vi "shuttercontrol.vi"(1 "error in":errorcluster, 2 "command":string) -> (0 "error out":errorcluster)   [LabVIEW 2015]
uses:
  <vilib>/DAQmx/write.llb/DAQmx Write (Digital Bool 1Line 1Point).vi
  <vilib>/DAQmx/create/channels.llb/DAQmx Create Channel (DO-Digital Output).vi
  <vilib>/DAQmx/miscellaneous.llb/DAQmx Fill In Error Info.vi
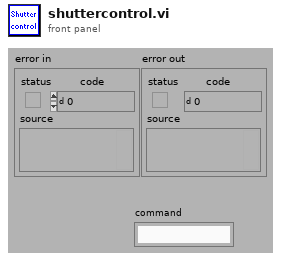
[diagram p1: front panel]
types:
  T1 = typedef "XYZStage.lvlib/XYZStage Configuration.ctl" = cluster{"VISA resource name":refnum<visa-resource-name>, "Timeout (3sec)":u32}
  T2 = cluster{"StageS":i32, "StageL":i32, "currmeas data dir":path, "image OD":u16, "contour OD":u16, "point OD":u16, "AOlines":tag[], "AIlines":tag[], "CI lines":tag[], "DO lines":tag[], "AO names":string[], "CI names":string[], "AI names":string[], "DO names":string[], "CIextensions":string[], "AIextensions":string[], "Voltage to Ygalvo":i32, "Voltage to Xgalvo":i32, "Voltage to patch":i32, "640 shutter":i32, "2P shutter":i32, "LT timestamp":u32, "Vp":i32, "Ip":i32, "camera trigger":i32, "master data dir":path, "voltage to Zpos":i32, "Vto2P":i32, "640 AO":i32, "488 AO":i32, "532 AO":i32, "640TTL":u32, "488TTL":u32, "532TTL":u32, "Device 1 sampleclock out":tag, "Device 1 Starttrigger out":tag, "Device 2 sampleclock in":tag, "Device 2 StartTrigger in ":tag, "2PODTTL":u32, "488 shutter":u32, "LCVR red":u32, "LCVR blue":u32, "Sutter Stage Config":T1}
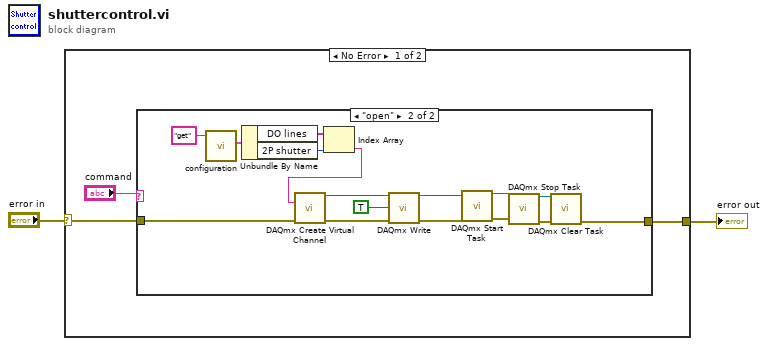
[diagram p0: block diagram]
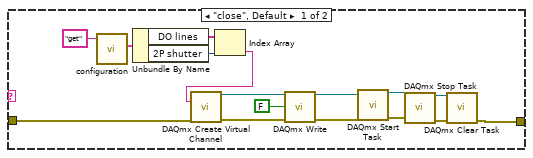
[diagram p2: hidden frame]
diagram:
  n1 = case shown="No Error" "error in" {
    selector: "error in" -> [w4 w38]
    tunnel: [w3 w38] -> w1
    frame No Error {
      n2 = case shown="\"open\"" "command" {
        tunnel: w4 -> [w12 w29]
        tunnel: [w11 w28] -> w3
        frame "close", Default {
          n3 = call "configuration.vi"("command"="get") -> ("config out"=w9:T2)  [unwired: 2 in, 1 out]
          n4 = Unbundle By Name(w9) -> ("DO lines"=w8:tag[], "2P shutter"=w6:i32)
          n5 = Index Array(array=w8, index=w6) -> (element=w7:tag)
          n6 = call-poly <vilib>:"DAQmx Create Virtual Channel.vi"("lines"=w7, "error in"=w12) -> ("task out"=w15:refnum<k21>, "error out"=w14:errorcluster)  [unwired: 12 in]
          n7 = call-poly <vilib>:"DAQmx Write.vi"("task/channels in"=w15, "data"=FALSE, "error in"=w14) -> ("task out"=w16:refnum<k21>, "error out"=w17:errorcluster)  [unwired: 10 in, 1 out]
          n8 = call <vilib>:"DAQmx Start Task.vi"("task/channels in"=w16, "error in"=w17) -> ("task out"=w18:refnum<k21>, "error out"=w19:errorcluster)  [unwired: 12 in]
          n9 = call <vilib>:"DAQmx Stop Task.vi"("task/channels in"=w18, "error in"=w19) -> ("task out"=w20:refnum<k21>, "error out"=w21:errorcluster)  [unwired: 12 in]
          n10 = call <vilib>:"DAQmx Clear Task.vi"("task in"=w20, "error in"=w21) -> ("error out"=w11:errorcluster)  [unwired: 13 in]
        }
        frame "open" {
          n11 = call "configuration.vi"("command"="get") -> ("config out"=w25:T2)  [unwired: 2 in, 1 out]
          n12 = Unbundle By Name(w25) -> ("DO lines"=w24:tag[], "2P shutter"=w22:i32)
          n13 = Index Array(array=w24, index=w22) -> (element=w23:tag)
          n14 = call-poly <vilib>:"DAQmx Create Virtual Channel.vi"("lines"=w23, "error in"=w29) -> ("task out"=w31:refnum<k21>, "error out"=w30:errorcluster)  [unwired: 12 in]
          n15 = call-poly <vilib>:"DAQmx Write.vi"("task/channels in"=w31, "data"=TRUE, "error in"=w30) -> ("task out"=w32:refnum<k21>, "error out"=w33:errorcluster)  [unwired: 10 in, 1 out]
          n16 = call <vilib>:"DAQmx Start Task.vi"("task/channels in"=w32, "error in"=w33) -> ("task out"=w34:refnum<k21>, "error out"=w35:errorcluster)  [unwired: 12 in]
          n17 = call <vilib>:"DAQmx Stop Task.vi"("task/channels in"=w34, "error in"=w35) -> ("task out"=w36:refnum<k21>, "error out"=w37:errorcluster)  [unwired: 12 in]
          n18 = call <vilib>:"DAQmx Clear Task.vi"("task in"=w36, "error in"=w37) -> ("error out"=w28:errorcluster)  [unwired: 13 in]
        }
      }
    }
    frame Error {
    }
  }
  "error out" <- w1
